vi "Apply and Get Shutter State.vi"(10 "Data Cluster":T1, 11 "Shutter State":T2=enum."Open") -> (0 "error out":errorcluster, 2 "plState":i32, 3 "SC_GetOPState":i32)   [LabVIEW 2020, in "Shutter.lvlib"]
uses:
  Shutter.lvlib
  Shutter State.ctl
  Module Data--cluster.ctl
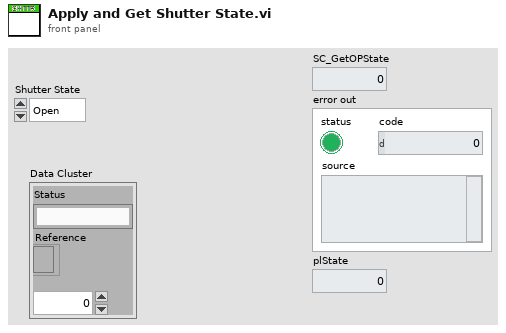
[diagram p1: front panel]
types:
  T1 = typedef "Shutter.lvlib/Module Data--cluster.ctl" = cluster{"Status":string, "Reference":refnum<k7>, "plState":i32}
  T2 = typedef "Shutter State.ctl" = enum16{"None", "Open", "Closed"}
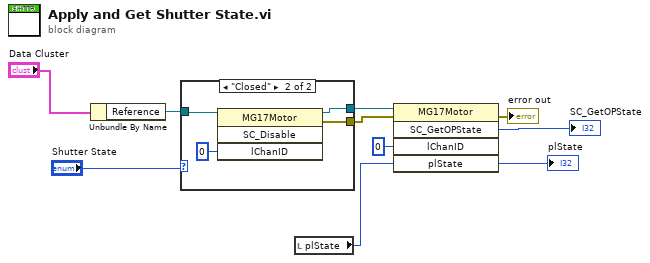
[diagram p0: block diagram]
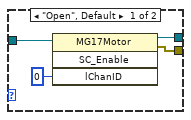
[diagram p2: hidden frame]
diagram:
  n1 = Unbundle By Name("Data Cluster") -> ("Reference"=w9:refnum<k7>)
  n2 = case shown="\"Closed\"" "Shutter State" {
    tunnel: w9 -> [w14 w18]
    tunnel: [w13 w17] -> w8
    tunnel: [w11 w16] -> w6
    frame "Open", Default {
      n3 = invoke class="MG17Motor" method="SC_Enable"(reference=w14, "lChanID"=0) -> (reference out=w13:refnum<k7>, error out=w11:errorcluster)  [unwired: 2 in, 2 out]
    }
    frame "Closed" {
      n4 = invoke class="MG17Motor" method="SC_Disable"(reference=w18, "lChanID"=0) -> (reference out=w17:refnum<k7>, error out=w16:errorcluster)  [unwired: 2 in, 2 out]
    }
  }
  n5 = local read "plState"() -> (w1:i32)
  n6 = invoke class="MG17Motor" method="SC_GetOPState"(reference=w8, error in=w6, "lChanID"=0, "plState"=w1) -> (error out=→"error out":errorcluster, "SC_GetOPState"=→"SC_GetOPState":i32, "plState"=→"plState":i32)  [unwired: 1 in, 2 out]
